vi "Write Sampling clock.vi"(8 "error in (no error)":errorcluster, 10 "Sampling clock":T1, 11 "RP Instrument in":refnum<class "RP Instrument.lvclass">) -> (0 "error out":errorcluster, 3 "RP Instrument out":refnum<class "RP Instrument.lvclass">)   [LabVIEW 2020, in "RP Instrument.lvclass"]
uses:
  RP Instrument.lvclass
  RP Instrument.lvclass/RP Instrument.ctl
  Controls/Sampling clock.ctl
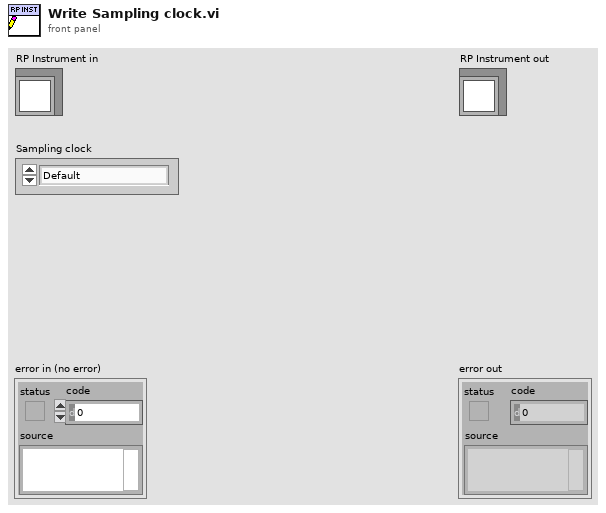
[diagram p1: front panel]
types:
  T1 = typedef "Sampling clock.ctl" = enum16{"Default", "Internal", "Extention connector", "Programmable logic"}
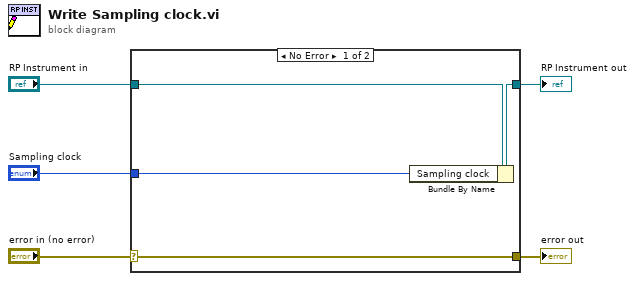
[diagram p0: block diagram]
diagram:
  n1 = case shown="No Error" "error in (no error)" {
    selector: "error in (no error)" -> [w9 w10]
    tunnel: [w9 w10] -> w4
    tunnel: [w7 w11] -> w2
    tunnel: "RP Instrument in" -> [w8 w11]
    tunnel: "Sampling clock" -> [w6 _]
    frame No Error {
      n2 = Bundle By Name(cluster=w8, "Sampling clock"=w6) -> (w7:refnum<class "RP Instrument.lvclass">)
    }
    frame Error {
    }
  }
  "error out" <- w4
  "RP Instrument out" <- w2
